vi "RSZVB Calibration Auto Type.vi"(0 "VISA session":refnum<visa-resource-name>, 1 "Channel (1)":i32=1, 2 "Parameters (2: Full One Port)":i32(ring)=2 items=["Full One Port"=2, "One Path Two Port"=4, "Full N-port"=10, "Separate Full Two-Port"=11], 3 "Calibration Kit Name":string, 4 "Analyzer Port 1 (1)":i32=1, 5 "error in (no error)":errorcluster {"code" format="%.0x"}, 6 "Analyzer Port 3 (0)":i32, 7 "Analyzer Port 4 (0)":i32, 8 "Cal Unit Port 1 (1)":i32=1, 9 "Cal Unit Port 2 (0)":i32, 10 "Cal Unit Port 3 (0)":i32, 11 "Cal Unit Port 4 (0)":i32, 12 "Analyzer Port 2 (0)":i32) -> (14 "dup VISA session":refnum<visa-resource-name>, 19 "error out":errorcluster {"code" format="%.0x"})   [LabVIEW 2011]
doc: "This VI selects and initiates a one-port, two-port, three-port or four-port automatic calibration at arbitrary analyzer and calibration unit ports.\n\nNote(s):\n\n(1) Port numbers of the analyzer:\nFor an n-port automatic calibration (n = 1 to 4), n arbitrary (not necessarily consecutive) port numbers must be specified.\n\n(2) Port numbers of the cal unit:\nFor an n-port automatic calibration (n = 1 to 4), n arbitrary (not necessarily consecutive) port numbers must be specified. It is possible to combine arbitrary (not necessarily matching) pairs of analyzer and cal unit ports.\n \nRemote-control command(s):\n[SENSe<Ch>:]CORRection:COLLect:AUTO:PORTs:TYPE <cal_type>,'<file_name>',<analyzer_port_no>,<cal_unit_port_no>{,<analyzer_port_no>,<cal_unit_port_no>}"
uses:
  _utility/RSZVB Global Data.vi
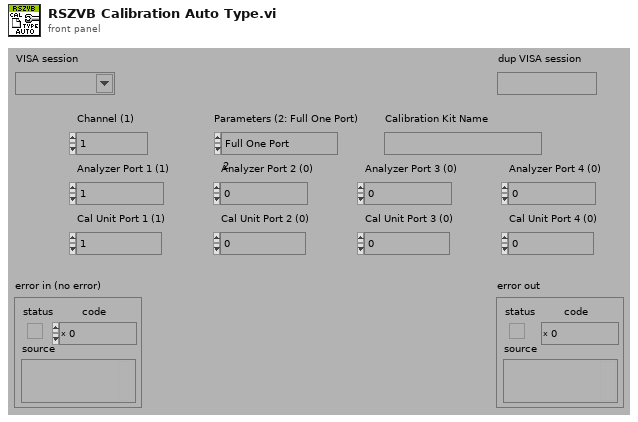
[diagram p1: front panel]
types:
  T1 = cluster{"Error Checking (T: On)":bool, "Installed Options":string[], "Data Valid?":bool, "Ports":i32, "Model":string[], "Option Checking (T: On)":bool}[]
  T2 = cluster{"Error Checking (T: On)":bool, "Installed Options":string[], "Data Valid?":bool, "Ports":i32, "Model":string[], "Option Checking (T: On)":bool}
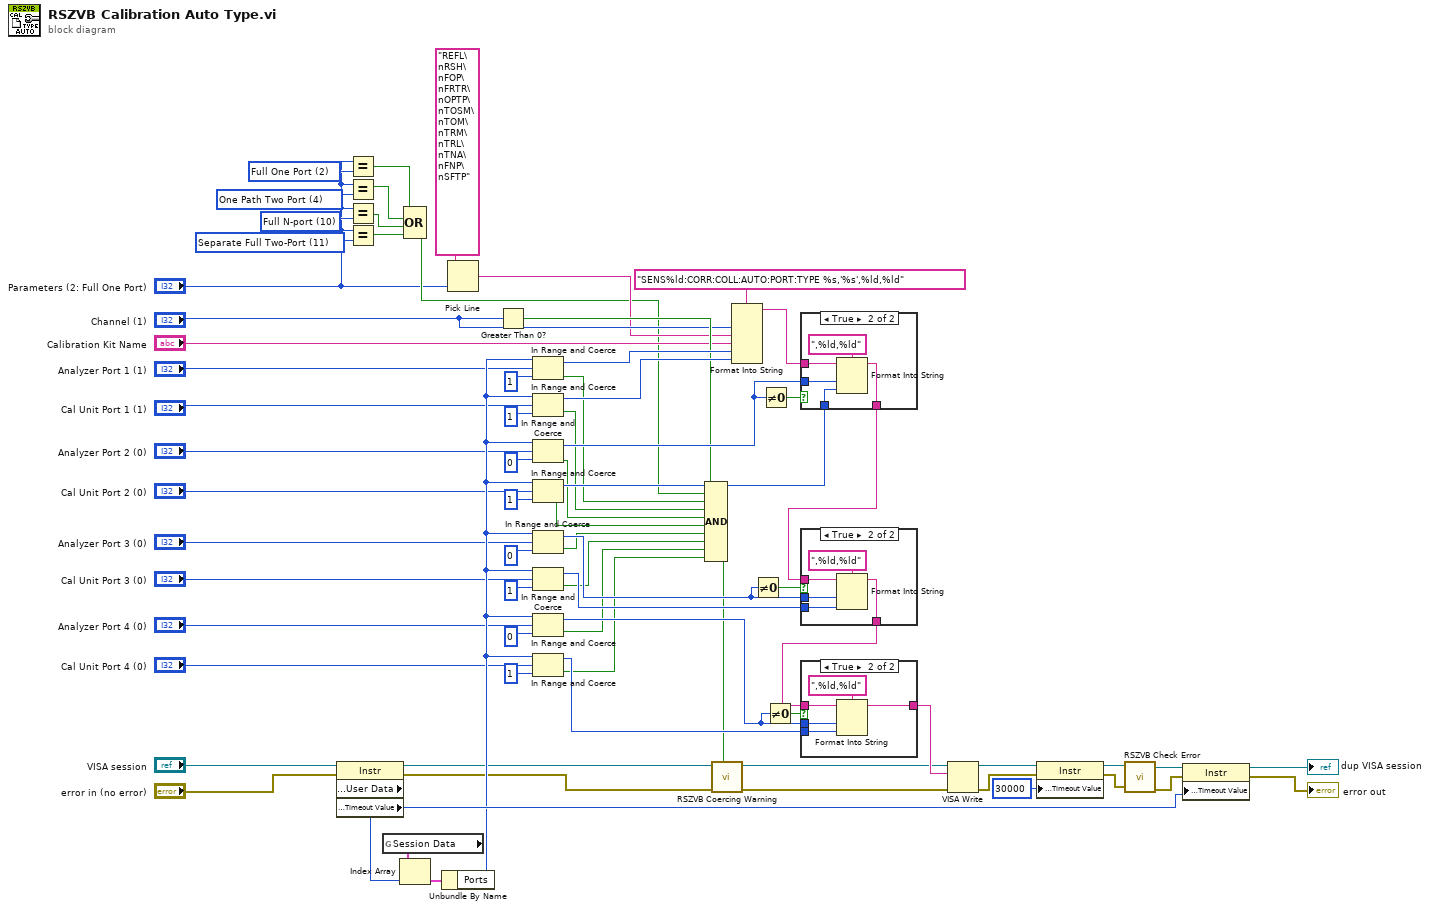
[diagram p0: block diagram]
diagram:
  w10 = 11 items=["Full One Port"=2, "One Path Two Port"=4, "Full N-port"=10, "Separate Full Two-Port"=11] ("Parameters (2: Full One Port)")
  w9 = 10 items=["Full One Port"=2, "One Path Two Port"=4, "Full N-port"=10, "Separate Full Two-Port"=11] ("Parameters (2: Full One Port)")
  w8 = 4 items=["Full One Port"=2, "One Path Two Port"=4, "Full N-port"=10, "Separate Full Two-Port"=11] ("Parameters (2: Full One Port)")
  w7 = 2 items=["Full One Port"=2, "One Path Two Port"=4, "Full N-port"=10, "Separate Full Two-Port"=11] ("Parameters (2: Full One Port)")
  n1 = property class="Instr"(reference="VISA session", error in="error in (no error)") -> (reference out=w36:refnum<visa-resource-name>, error out=w35:errorcluster, "General Settings:User Data"=w34:u32, "General Settings:Timeout Value"=w70:u32)
  n2 = Equal?(x="Parameters (2: Full One Port)", y=w7) -> (x = y?=w6:bool)
  n3 = Equal?(x="Parameters (2: Full One Port)", y=w8) -> (x = y?=w5:bool)
  n4 = Equal?(x="Parameters (2: Full One Port)", y=w9) -> (x = y?=w4:bool)
  n5 = Equal?(x="Parameters (2: Full One Port)", y=w10) -> (x = y?=w3:bool)
  n6 = global read "RSZVB Global Data.vi" "Session Data"() -> (w33:T1)
  n7 = Index Array(array=w33, index=w34) -> (element=w32:T2)
  n8 = Compound Arithmetic op=OR(w6, w5, w4, w3) -> (w2:bool)
  n9 = Unbundle By Name(w32) -> ("Ports"=w59:i32)
  n10 = Pick Line(multi-line string="REFL\nRSH\nFOP\nFRTR\nOPTP\nTOSM\nTOM\nTRM\nTRL\nTNA\nFNP\nSFTP", line index="Parameters (2: Full One Port)") -> (output string=w11:string)  [unwired: 1 in]
  n11 = Greater Than 0?(x="Channel (1)") -> (x > 0?=w31:bool)
  n12 = In Range and Coerce(upper limit=w59, x="Analyzer Port 1 (1)", lower limit=1) -> (coerced(x)=w52:i32, In Range?=w40:bool)
  n13 = In Range and Coerce(upper limit=w59, x="Cal Unit Port 1 (1)", lower limit=1) -> (coerced(x)=w62:i32, In Range?=w41:bool)
  n14 = In Range and Coerce(upper limit=w59, x="Analyzer Port 2 (0)", lower limit=0) -> (coerced(x)=w63:i32, In Range?=w42:bool)
  n15 = In Range and Coerce(upper limit=w59, x="Cal Unit Port 2 (0)", lower limit=1) -> (coerced(x)=w64:i32, In Range?=w43:bool)
  n16 = In Range and Coerce(upper limit=w59, x="Analyzer Port 3 (0)", lower limit=0) -> (coerced(x)=w67:i32, In Range?=w54:bool)
  n17 = In Range and Coerce(upper limit=w59, x="Cal Unit Port 3 (0)", lower limit=1) -> (coerced(x)=w65:i32, In Range?=w55:bool)
  n18 = In Range and Coerce(upper limit=w59, x="Analyzer Port 4 (0)", lower limit=0) -> (coerced(x)=w68:i32, In Range?=w56:bool)
  n19 = In Range and Coerce(upper limit=w59, x="Cal Unit Port 4 (0)", lower limit=1) -> (coerced(x)=w66:i32, In Range?=w57:bool)
  n20 = Compound Arithmetic op=AND(w31, w2, w40, w41, w42, w43, w54, w55, w56, w57) -> (w30:bool)
  n21 = call "RSZVB Coercing Warning.vi"("In Range?"=w30, "error in (no error)"=w35, "VISA session"=w36) -> ("error out"=w29:errorcluster, "dup VISA session"=w28:refnum<visa-resource-name>)  [unwired: 7 in]
  n22 = Format Into String(format string="SENS%ld:CORR:COLL:AUTO:PORT:TYPE %s,'%s',%ld,%ld", "Channel (1)", w11, "Calibration Kit Name", w52, w62) -> (resulting string=w46:string)  [unwired: 2 in, 1 out]
  n23 = Not Equal To 0?(x=w67) -> (x != 0?=w47:bool)
  n24 = Not Equal To 0?(x=w63) -> (x != 0?=w45:bool)
  n25 = Not Equal To 0?(x=w68) -> (x != 0?=w49:bool)
  n26 = case shown="True" w45 {
    tunnel: w46 -> [w77 w82]
    tunnel: w63 -> [_ w80]
    tunnel: [w77 w79] -> w48
    tunnel: w64 -> [_ w78]
    frame False {
    }
    frame True {
      n27 = Format Into String(format string=",%ld,%ld", initial string=w82, w80, w78) -> (resulting string=w79:string)  [unwired: 1 in, 1 out]
    }
  }
  n28 = case shown="True" w47 {
    tunnel: w48 -> [w83 w88]
    tunnel: w67 -> [_ w86]
    tunnel: [w83 w85] -> w50
    tunnel: w65 -> [_ w84]
    frame False {
    }
    frame True {
      n29 = Format Into String(format string=",%ld,%ld", initial string=w88, w86, w84) -> (resulting string=w85:string)  [unwired: 1 in, 1 out]
    }
  }
  n30 = case shown="True" w49 {
    tunnel: w50 -> [w89 w94]
    tunnel: w68 -> [_ w92]
    tunnel: [w89 w91] -> w51
    tunnel: w66 -> [_ w90]
    frame False {
    }
    frame True {
      n31 = Format Into String(format string=",%ld,%ld", initial string=w94, w92, w90) -> (resulting string=w91:string)  [unwired: 1 in, 1 out]
    }
  }
  n32 = VISA Write(VISA resource name=w28, write buffer=w51, error in (no error)=w29) -> (VISA resource name out=w74:refnum<visa-resource-name>, error out=w75:errorcluster)  [unwired: 1 out]
  n33 = property class="Instr"(reference=w74, error in=w75, "General Settings:Timeout Value"=u32 30000) -> (reference out=w73:refnum<visa-resource-name>, error out=w76:errorcluster)
  n34 = call "RSZVB Check Error.vi"("error in (no error)"=w76, "VISA session"=w73) -> ("error out"=w71:errorcluster, "dup VISA session"=w72:refnum<visa-resource-name>)  [unwired: 8 in]
  n35 = property class="Instr"(reference=w72, error in=w71, "General Settings:Timeout Value"=w70) -> (reference out=→"dup VISA session":refnum<visa-resource-name>, error out=→"error out":errorcluster)
